vi "Get Recent Articles.vi"(8 "error in (no error)":errorcluster, 10 "how many":i32=4, 11 "Feed in":refnum<class "Feed.lvclass">) -> (0 "error out":errorcluster, 2 "recent articles":string[](array[string]), 3 "Feed out":refnum<class "Feed.lvclass">)   [LabVIEW 2020, in "Feed.lvclass"]
uses:
  <vilib>/NI_RSS/Feed/Feed.lvclass
  <vilib>/NI_RSS/FeedItem/FeedItem.lvclass
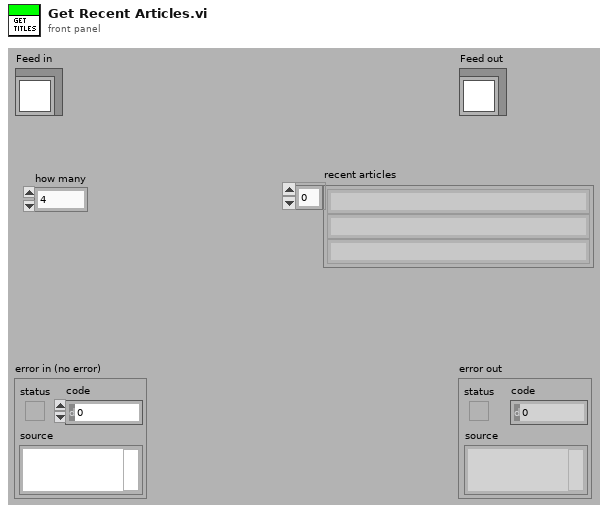
[diagram p1: front panel]
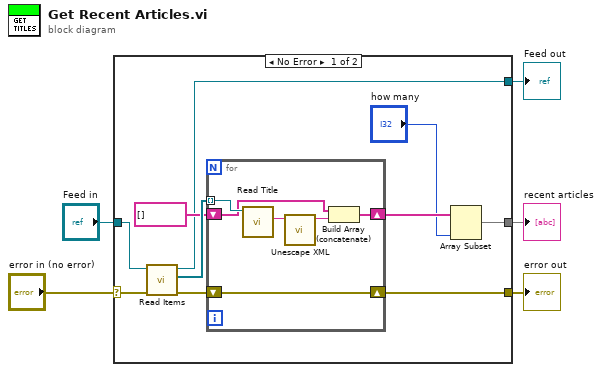
[diagram p0: block diagram]
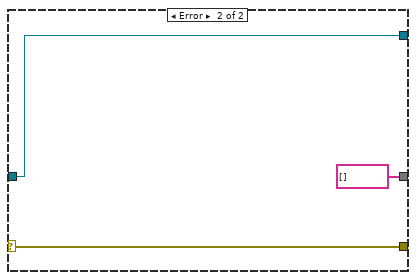
[diagram p2: hidden frame]
diagram:
  n1 = case shown="No Error" "error in (no error)" {
    selector: "error in (no error)" -> [w9 w24]
    tunnel: [w7 w24] -> w4
    tunnel: [w6 w23] -> w2
    tunnel: "Feed in" -> [w15 w23]
    tunnel: [w11 string[] []] -> w1
    frame No Error {
      n2 = call-dynamic "Read Items.vi"("error in (no error)"=w9, "Feed.lvclass in"=w15) -> ("error out"=w8:errorcluster, "Items"=w14:refnum<class "FeedItem.lvclass">[], "Feed.lvclass out"=w6:refnum<class "Feed.lvclass">)  [unwired: 1 in, 6 out]
      n3 = for {
        tunnel: w14 -> [w21] mode=indexing
        shift-right: [w20] -> w12
        shift-left: string[] [] -> [w19]
        shift-right: [w16] -> w7
        shift-left: w8 -> [w16]
        n4 = call-dynamic "Read Title.vi"("FeedItem.lvclass in"=w21) -> ("Title"=w18:string)  [unwired: 1 in, 9 out]
        n5 = call <vilib>:"Unescape XML.vi"("XML String In"=w18) -> ("XML String Out"=w17:string)  [unwired: 9 in, 1 out]
        n6 = Build Array (concatenate)(w19, w17) -> (w20:string[])
      }
      n7 = Array Subset(array=w12, length="how many") -> (w11:string[])  [unwired: 1 in]
    }
    frame Error {
    }
  }
  "error out" <- w4
  "Feed out" <- w2
  "recent articles" <- w1
